vi "Image Load.vi"(8 "error in":errorcluster, 11 "File":string="c:\\temp\\hello.bmp") -> (0 "error out":errorcluster, 3 "Surface Pointer":u32 format="%.0x")   [LabVIEW 2015, in "LibSDL2_Image.lvlib"]
uses:
  LibSDL2_Image.lvlib
  LibSDL2 Wrapper/DLL/SDL2_image.dll
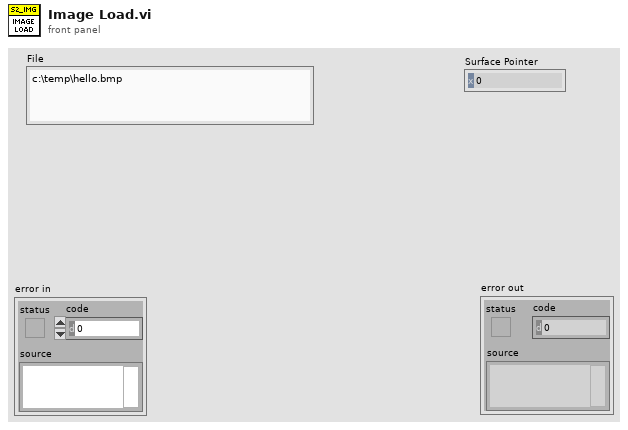
[diagram p1: front panel]
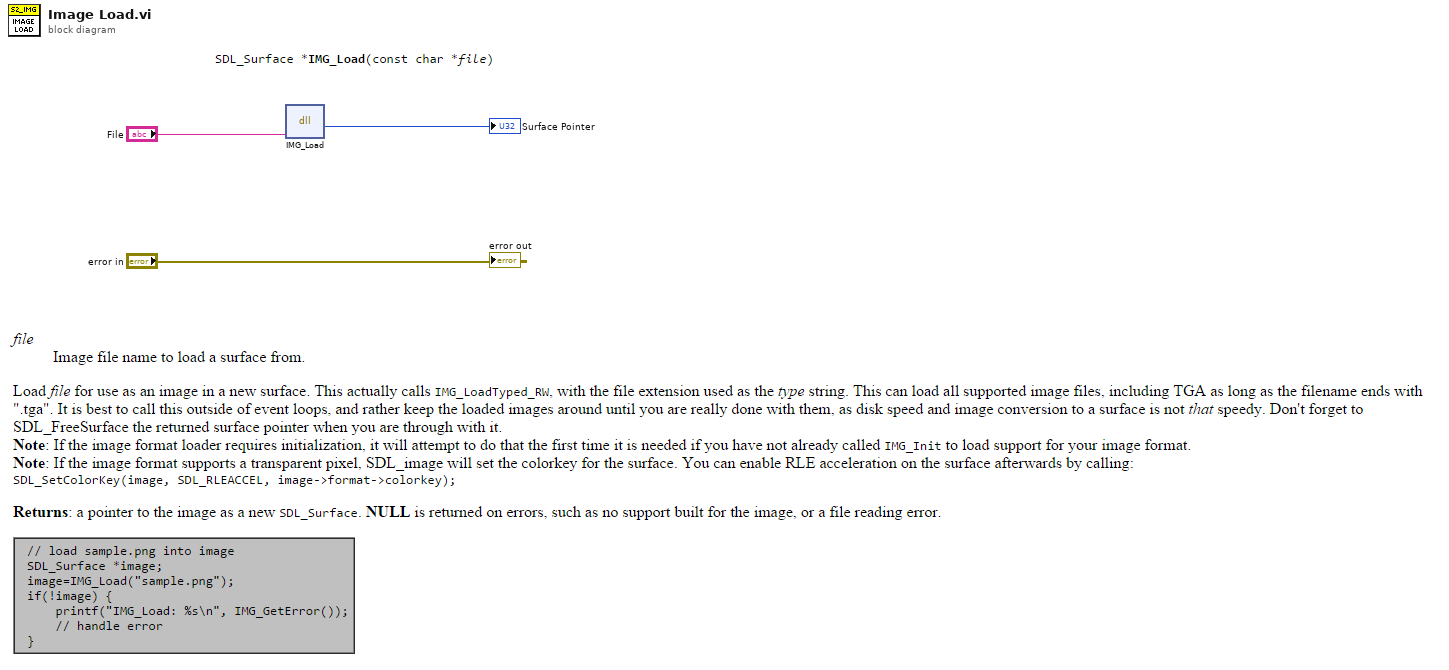
[diagram p0: block diagram]
diagram:
  n1 = dll-call lib="C:/dev/PGS/LabSDL2/Source/Libraries/LibSDL2 Wrapper/DLL/SDL2_image.dll" fn="IMG_Load"("file"="File") -> ("return type"=→"Surface Pointer":u32)  [unwired: 4 in, 2 out]
  "error out" <- "error in"
